vi "并联IT6332B.vi"(8 "error in (no error)":errorcluster, 11 "VISA resource name":refnum<visa-resource-name>) -> (0 "错误输出":errorcluster, 3 "VISA资源名称输出":refnum<visa-resource-name>)   [LabVIEW 2021]
uses:
  <instrlib>/IT6300/IT6300.lvlib
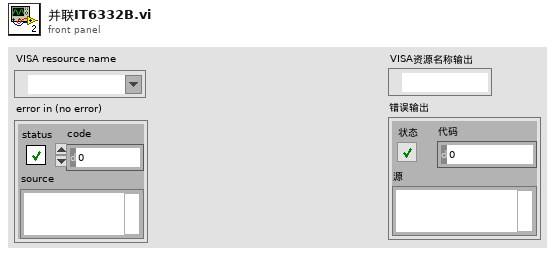
[diagram p1: front panel]
types:
  T1 = cluster{"Channel1":bool, "Channel2":bool, "Channel3":bool}
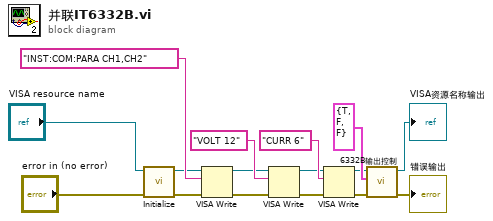
[diagram p0: block diagram]
diagram:
  n1 = call <instrlib>:"Initialize.vi"("error in (no error)"="error in (no error)", "VISA resource name"="VISA resource name") -> ("error out"=w10:errorcluster, "VISA resource name out"=w9:refnum<visa-resource-name>)  [unwired: 8 in]
  n2 = VISA Write(VISA resource name=w9, write buffer="INST:COM:PARA CH1,CH2" ("写入缓冲区"), error in (no error)=w10) -> (VISA resource name out=w6:refnum<visa-resource-name>, error out=w1:errorcluster)  [unwired: 1 out]
  n3 = VISA Write(VISA resource name=w6, write buffer="VOLT 12" ("写入缓冲区"), error in (no error)=w1) -> (VISA resource name out=w5:refnum<visa-resource-name>, error out=w2:errorcluster)  [unwired: 1 out]
  n4 = VISA Write(VISA resource name=w5, write buffer="CURR 6" ("写入缓冲区"), error in (no error)=w2) -> (VISA resource name out=w4:refnum<visa-resource-name>, error out=w3:errorcluster)  [unwired: 1 out]
  n5 = call "6332B输出控制.vi"("错误输入"=w3, "Choose Channel"=T1 {"Channel1"=TRUE, "Channel2"=FALSE, "Channel3"=FALSE}, "VISA资源名称"=w4) -> ("错误输出"=→"错误输出":errorcluster, "VISA资源名称输出"=→"VISA资源名称输出":refnum<visa-resource-name>)  [unwired: 7 in]
